vi "Get Plugins from Configuration.vi"(8 "error in (no error)":errorcluster, 11 "Application Data In":T2) -> (0 "error out":errorcluster, 1 "Settings Items":T1[](array[typedef]), 2 "Plugin Items":T1[](array[typedef]), 3 "Application Data out":T2)   [LabVIEW 2019, in "DSF Configuration Utility.lvlib"]
uses:
  DSF Configuration Utility.lvlib
  ID to Tree Items/Tree Item Type.ctl
  VeriStand/Data Sharing Custom Device/Source/DSF Core.lvlibp/Classes/Configuration Session/Configuration Session.lvclass
  Main VI/Application Data.ctl
  Tree Item.ctl
  Main VI/View Mode.ctl
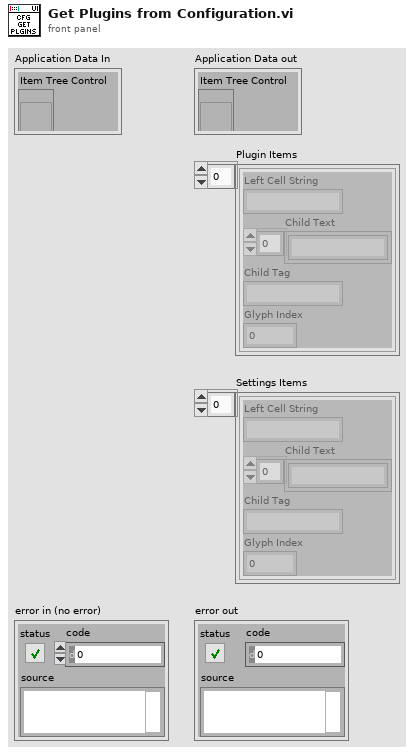
[diagram p1: front panel]
types:
  T1 = typedef "DSF Configuration Utility.lvlib/Tree Item.ctl" = cluster{"Left Cell String":string, "Child Text":string[], "Child Tag":string, "Glyph Index":i32}
  T2 = typedef "DSF Configuration Utility.lvlib/Application Data.ctl" = cluster{"Item Tree Control":refnum<vi>, "Value Tree Control":refnum<vi>, "Configuration Session":refnum<class "Configuration Session.lvclass">, "Top-Level VI":refnum<vi>, "View State":T3, "menu reference":refnum<k9>}
  T3 = typedef "DSF Configuration Utility.lvlib/View Mode.ctl" = enum16{"Tree", "List"}
  T4 = typedef "DSF Core.lvlibp/DSF Engine Plugin Configuration.ctl" = cluster{"name":string, "components":string[], "cycle timing":T5, "threads":T6[], "transfer groups":T8[], "settings":T7}
  T5 = typedef "DSF Core.lvlibp/DSF Timing Info.ctl" = cluster{"priority":u64, "decimation":u64, "offset":u64}
  T6 = typedef "DSF Core.lvlibp/DSF Engine Plugin Thread Configuration.ctl" = cluster{"processor":i32, "priority offset":i16, "settings":T7}
  T7 = typedef "DSF Core.lvlibp/DSF Settings Info.ctl" = cluster{"component":string, "name":string, "values":cluster{"key":string, "value":string}[]}[]
  T8 = typedef "DSF Core.lvlibp/DSF Engine Transfer Group Configuration.ctl" = cluster{"name":string, "direction":T9, "cycle timing":T5, "thread index":i32, "settings":T7, "transfers":T10[], "timeout behavior":T14}
  T9 = typedef "DSF Core.lvlibp/DSF Direction.ctl" = enum8{"Tx", "Rx"}
  T10 = typedef "DSF Core.lvlibp/DSF Engine Transfer Configuration.ctl" = cluster{"name":string, "byte order":T11, "settings":T7, "channels":T12[]}
  T11 = typedef "DSF Core.lvlibp/DSF Byte Order.ctl" = enum8{"big-endian", "little-endian"}
  T12 = typedef "DSF Core.lvlibp/DSF Engine Channel Configuration.ctl" = cluster{"string offset":u64, "name":string, "units":string, "engine data type":T13, "string data type":T13, "settings":T7}
  T13 = typedef "DSF Core.lvlibp/DSF Data Type.ctl" = enum8{"Bool", "SGL", "DBL", "I8", "I16", "I32", "I64", "U8", "U16", "U32", "U64"}
  T14 = typedef "DSF Core.lvlibp/DSF Timeout Behavior.ctl" = enum8{"Increment Late Count", "Throw Error"}
  T15 = typedef "DSF Configuration Utility.lvlib/Tree Item Type.ctl" = enum16{"Plugin", "Group", "Transfer", "Channel", "Setting"}
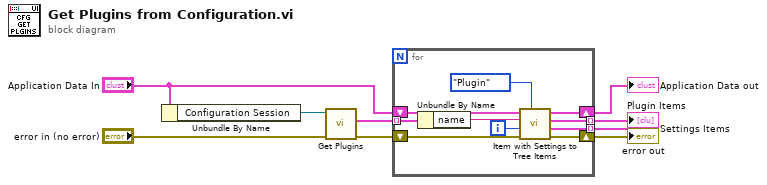
[diagram p0: block diagram]
diagram:
  n1 = Unbundle By Name("Application Data In") -> ("Configuration Session"=w5:refnum<class "Configuration Session.lvclass">)
  n2 = call "Get Plugins.vi"("error in (no error)"="error in (no error)", "configuration session in"=w5) -> ("error out"=w4:errorcluster, "plugins"=w3:T4[])  [unwired: 7 in, 1 out]
  n3 = for {
    tunnel: w3 -> [w16] mode=indexing
    tunnel: [w11] -> w8 mode=indexing
    tunnel: [w12] -> w7 mode=indexing
    shift-right: [w13] -> w9
    shift-left: w4 -> [w19]
    shift-right: [w10] -> w1
    shift-left: "Application Data In" -> [w18]
    i -> [w17]
    n4 = Unbundle By Name(w16) -> ("name"=w15:string)
    n5 = call "Item with Settings to Tree Items.vi"("item type"=Tree_Item_Type."Plugin", "error in (no error)"=w19, "item index"=w17, "item name"=w15, "Application Data in"=w18) -> ("error out"=w13:errorcluster, "Settings Item"=w12:T1, "Item"=w11:T1, "Application Data out"=w10:T2)  [unwired: 3 in]
  }
  "Application Data out" <- w1
  "error out" <- w9
  "Plugin Items" <- w8
  "Settings Items" <- w7
